vi "TDT ET-Get Status.vi"(0 "TCP":T1, 7 "Timeout (ms)":i32=2000, 11 "error in (no error)":errorcluster) -> (15 "error out":errorcluster)   [LabVIEW 2015]
uses:
  Utility VIs/Type Defs/TCP Params.ctl
panel:
  out "Status":i32
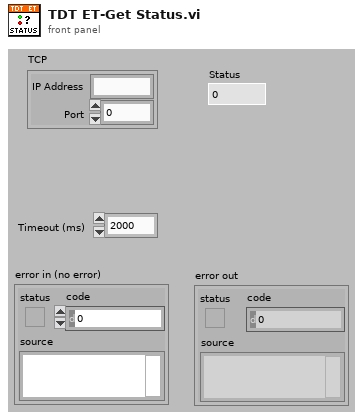
[diagram p1: front panel]
types:
  T1 = typedef "TCP Params.ctl" = cluster{"IP Address":string, "Port":i32}
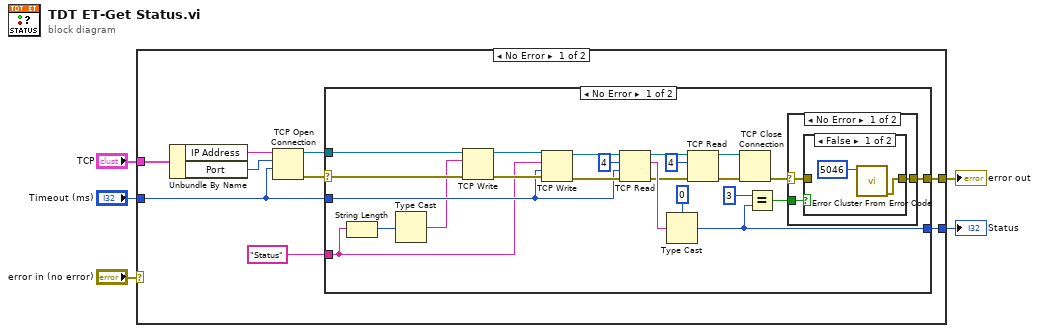
[diagram p0: block diagram]
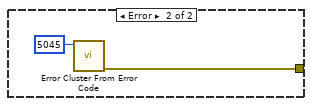
[diagram p4: hidden frame]
diagram:
  n1 = case shown="No Error" "error in (no error)" {
    selector: "error in (no error)" -> [_ w47]
    tunnel: [w8 w47] -> w4
    tunnel: "TCP" -> [w14 _]
    tunnel: "Timeout (ms)" -> [w9 _]
    tunnel: [w6 _] -> w1
    frame No Error {
      n2 = Unbundle By Name(w14) -> ("IP Address"=w7:string, "Port"=w13:i32)
      n3 = TCP Open Connection(address=w7, remote port or service name=w13, timeout ms (60000)=w9) -> (connection ID=w11:refnum<k5>, error out=w12:errorcluster)  [unwired: 2 in]
      n4 = case shown="No Error" w12 {
        selector: w12 -> [w30 _]
        tunnel: w11 -> [w29 _]
        tunnel: "Status" -> [w27 _]
        tunnel: w9 -> [w33 _]
        tunnel: [w15 w46] -> w8
        tunnel: [w18 _] -> w6
        frame No Error {
          n5 = String Length(string=w27) -> (length=w26:i32)
          n6 = Type Cast(x=w26) -> (*(type *) &x=w25:string)  [unwired: 1 in]
          n7 = TCP Write(connection ID=w29, data in=w25, error in (no error)=w30) -> (connection ID out=w28:refnum<k5>, error out=w37:errorcluster)  [unwired: 1 in, 1 out]
          n8 = TCP Write(connection ID=w28, data in=w27, error in (no error)=w37, 9:w33) -> (connection ID out=w35:refnum<k5>, error out=w36:errorcluster)  [unwired: 1 out]
          n9 = TCP Read(connection ID=w35, bytes to read=4, error in (no error)=w36, 9:w33) -> (connection ID out=w23:refnum<k5>, data out=w32:string, error out=w22:errorcluster)  [unwired: 1 in]
          n10 = Type Cast(type=0, x=w32) -> (*(type *) &x=w18:i32)
          n11 = TCP Read(connection ID=w23, bytes to read=4, error in (no error)=w22) -> (connection ID out=w20:refnum<k5>, error out=w21:errorcluster)  [unwired: 2 in, 1 out]
          n12 = TCP Close Connection(connection ID=w20, error in (no error)=w21) -> (error out=w19:errorcluster)  [unwired: 1 in, 1 out]
          n13 = Equal?(x=3, y=w18) -> (x = y?=w16:bool)
          n14 = case shown="No Error" w19 {
            selector: w19 -> [w39 w44]
            tunnel: w16 -> [w40 _]
            tunnel: [w38 w44] -> w15
            frame No Error {
              n15 = case shown="False" w40 {
                tunnel: w39 -> [_ w43]
                tunnel: [w42 w43] -> w38
                frame False {
                  n16 = call <vilib>:"Error Cluster From Error Code.vi"("error code (0)"=5046) -> ("error out"=w42:errorcluster)  [unwired: 8 in]
                }
                frame True {
                }
              }
            }
            frame Error {
            }
          }
        }
        frame Error {
          n17 = call <vilib>:"Error Cluster From Error Code.vi"("error code (0)"=5045) -> ("error out"=w46:errorcluster)  [unwired: 8 in]
        }
      }
    }
    frame Error {
    }
  }
  "error out" <- w4
  "Status" <- w1
